vi "MOSFET.vi"() -> ()   [LabVIEW 2016]
panel:
  in  "Stop Button":bool
  in  "Radio B":enum32{"I-T", "V-t", "R-t "}(radio)
  in  "CompliancetUnit":u16(ring)=2 items=["μA", "mA", "A"]
  in  "Compliance":sgl=0.1 min=0.1 max=1 step=0.1 format="%#.3f"
  in  "channel a 4":bool
  in  "channel a 3":bool
  in  "IV CLUS B 2":T1={"StartUnit"=1, "Voltage "=-10.0, "Timer"=0.1, "CompliancetUnit  2"=2} {"CompliancetUnit  2" items=["s"]; "Timer" min=0.1 max=1 step=0.1 format="%#.3f"; "StartUnit" items=["mV", "V"]; "Voltage" min=-20.0 max=20.0 step=0.001 format="%#.3f"}
  in  "channel a 2":bool
  in  "channel a":bool
  out "Chart 2":cluster{dbl[], dbl[]}[](graph)
  in  "Series 2600B":u16(ring)=5 items=["2602B  40V, 10A,100fA", "2604B  40V, 10A,100fA", "2612B  200V, 10A,100fA", "2614B  200V, 10A,100fA", "2634B  200V, 10A,1fA", "2636B  200V, 10A,0.1fA"]
  in  "IV CLUS B":T2={"B VolUnit"=1, "B Voltage"=-10.0, "Compliance B"=0.1, "CompliancetUnit B"=2} {"CompliancetUnit B" items=["μA", "mA", "A"]; "B VolUnit" items=["mV", "V"]; "B Voltage" min=-20.0 max=20.0 step=0.001 format="%#.3f"; "Compliance B" min=0.1 max=1 step=0.1 format="%#.3f"}
  in  "DataPoints":u32=21
  in  "IV CLUS":T3={"StepUnit"=1, "Step"=1.0, "StoptUnit"=1, "StartUnit"=1, "Stop"=10.0, "Start "=-10.0} {"StepUnit" items=["mV", "V"]; "Step" min=0.001 max=20.0 step=0.001 format="%#.3f"; "StoptUnit" items=["mV", "V"]; "StartUnit" items=["mV", "V"]; "Stop" min=-20.0 max=20.0 step=0.001 format="%#.3f"; "Start" min=-20.0 max=20.0 step=0.001 format="%#.3f"}
  in  "Save All":bool
  in  "SetOK":bool
  in  "Tab Control":T4(tab)
  out "Sheet":string[][](table)
  out "Sheet 2":string[][](table) caption="Sheet"
  out "Sheet 3":string[][](table) caption="Sheet"
  out "Sheet 4":string[][](table) caption="Sheet"
  out "Sheet 5":string[][](table) caption="Sheet"
  out "Sheet 6":string[][](table) caption="Sheet"
  out "Sheet 7":string[][](table) caption="Sheet"
  out "Sheet 8":string[][](table) caption="Sheet"
  out "Sheet 9":string[][](table) caption="Sheet"
  out "Sheet 10":string[][](table) caption="Sheet"
  out "Sheet 11":string[][](table) caption="Sheet"
  out "Sheet 12":string[][](table) caption="Sheet"
  out "Sheet 13":string[][](table) caption="Sheet"
  out "Sheet 14":string[][](table) caption="Sheet"
  out "Sheet 15":string[][](table) caption="Sheet"
  out "Sheet 16":string[][](table) caption="Sheet"
  out "Sheet 17":string[][](table) caption="Sheet"
  out "Sheet 18":string[][](table) caption="Sheet"
  out "Sheet 19":string[][](table) caption="Sheet"
  out "Sheet 20":string[][](table) caption="Sheet"
  out "Sheet 21":string[][](table) caption="Sheet"
  out "test time 2":string
  out "Chart":cluster{dbl[], dbl[]}[](graph)
  in  "Source Mode  (0: Voltage)":u16(ring) items=["Voltage", "Current"]
  out "TempChart":cluster{sgl[], dbl[]}[](array[cluster])
  out "AppArray":bool[](array[boolean])
  out "test time":timestamp
  out "RES":dbl
  in  "EXIT":bool
  # "Channel A"
  # "Channel B"
  # "PRCBE  2600B -MOSFET Test"
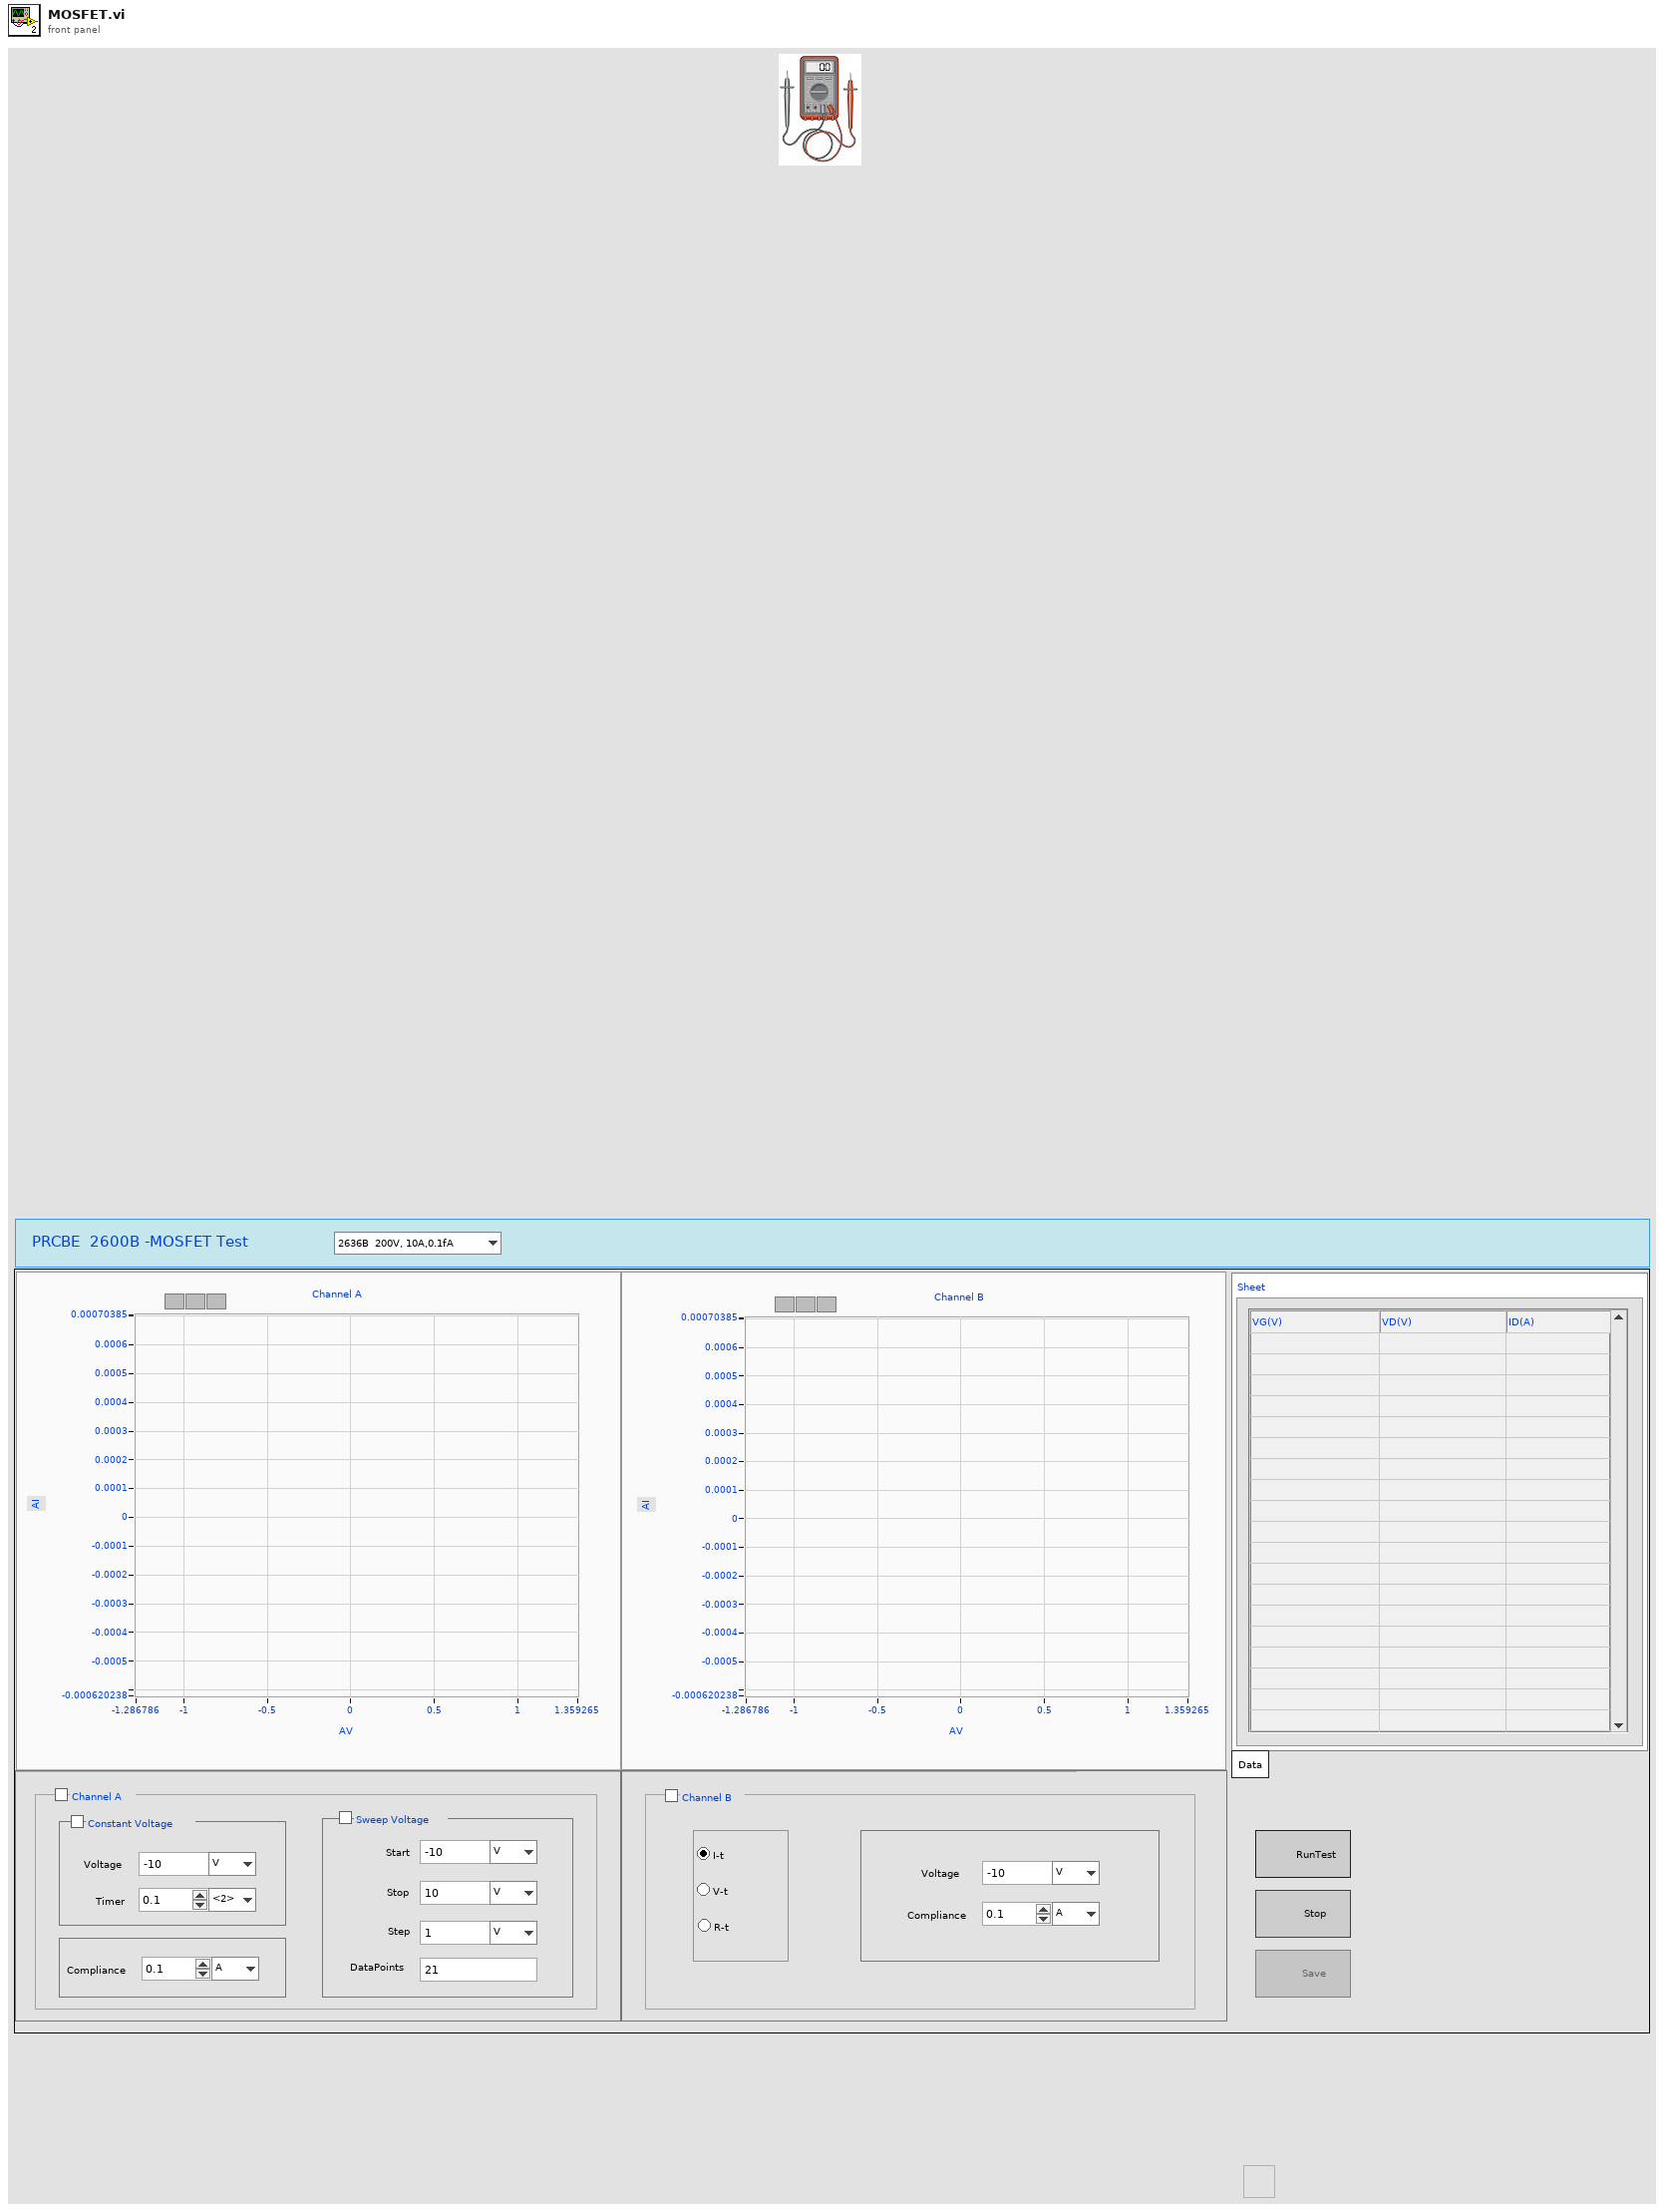
[diagram p1: front panel]
types:
  T1 = cluster{"StartUnit":u16, "Voltage ":dbl, "Timer":sgl, "CompliancetUnit  2":u16}
  T2 = cluster{"B VolUnit":u16, "B Voltage":dbl, "Compliance B":sgl, "CompliancetUnit B":u16}
  T3 = cluster{"StepUnit":u16, "Step":dbl, "StoptUnit":u16, "StartUnit":u16, "Stop":dbl, "Start ":dbl}
  T4 = enum32{"Data", "Append 1", "Append 2", "Append 3", "Append 4", "Append 5", "Append 6", "Append 7", "Append 8", "Append 9", "Append 10", "Append 11", "Append 12", "Append 13", "Append 14", "Append 15", "Append 16", "Append 17", "Append 18", "Append 19", "Append 20"}
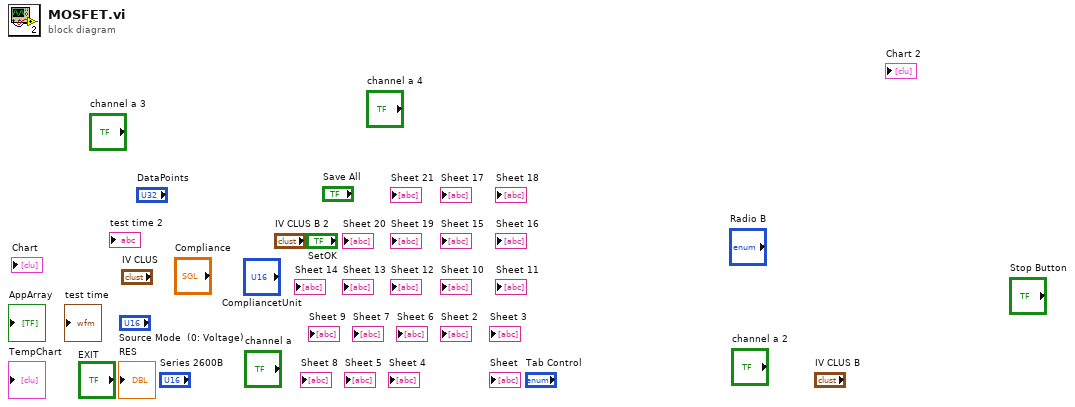
[diagram p0: block diagram]
diagram:
